vi "Process_single_meas.vi"(4 "Normalize?":bool, 6 "Calibration Constant (1/deg)":dbl, 7 "Magnet position":dbl, 8 "Magnetic Field (mT)":dbl, 9 "Actual Measurement":T2={"Elapsed Time (s)"=0.0, "Keithley"=0.0, "LockIn A"=[1.33515e-05, 1.14442e-05, 1.90736e-05, 41.634], "LockIn B"=[1.33515e-05, 1.14442e-05, 1.90736e-05, 41.634], "Dc intensity (V)"=0.0}) -> (3 "output cluster":T1)   [LabVIEW 2017]
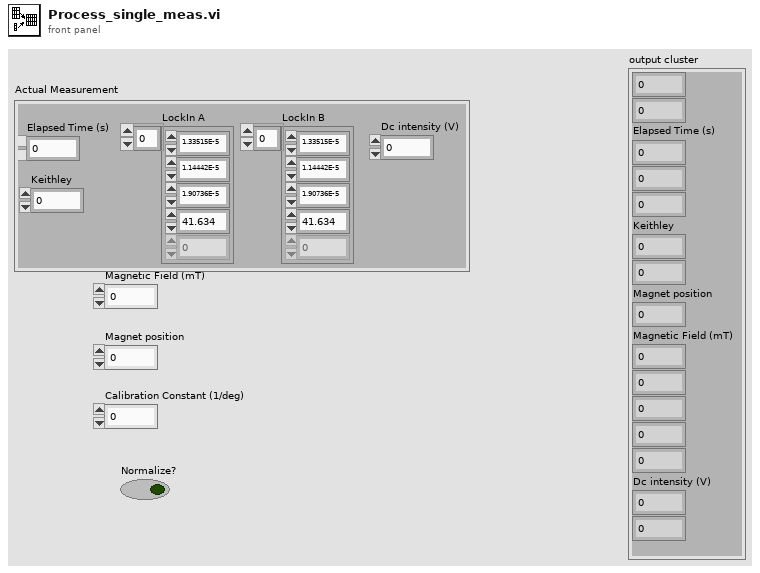
[diagram p1: front panel]
types:
  T1 = cluster{dbl, dbl, "Elapsed Time (s)":dbl, dbl, dbl, "Keithley":dbl, dbl, "Magnet position":dbl, "Magnetic Field (mT)":dbl, dbl, dbl, dbl, dbl, "Dc intensity (V)":dbl, dbl}
  T2 = cluster{"Elapsed Time (s)":dbl, "Keithley":dbl, "LockIn A":dbl[], "LockIn B":dbl[], "Dc intensity (V)":dbl}
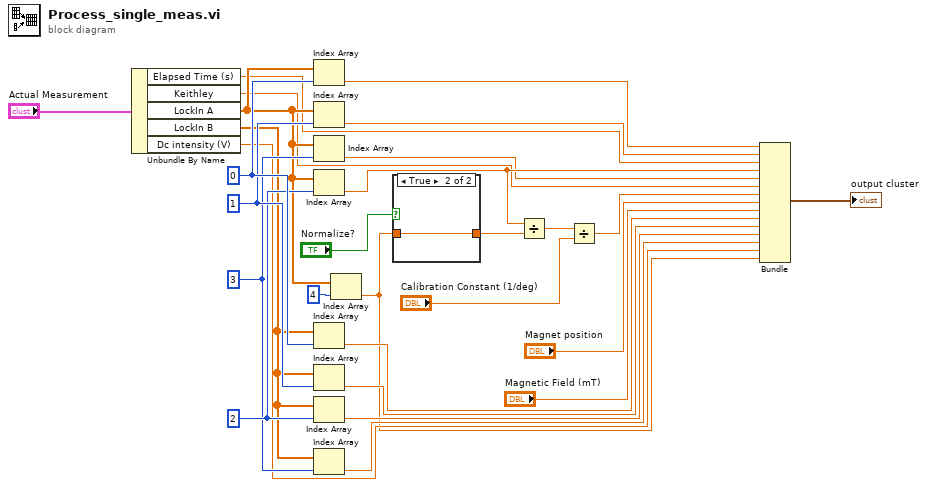
[diagram p0: block diagram]
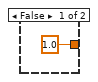
[diagram p2: hidden frame]
diagram:
  w23 = 3 ("index")
  w24 = 2 ("index")
  w25 = 1 ("index")
  w26 = 0 ("index")
  n1 = Unbundle By Name("Actual Measurement") -> ("Elapsed Time (s)"=w14:dbl, "Keithley"=w11:dbl, "LockIn A"=w19:dbl[], "LockIn B"=w22:dbl[], "Dc intensity (V)"=w3:dbl)
  n2 = Index Array(array=w19, index=w26) -> (element=w16:dbl)
  n3 = Index Array(array=w19, index=w25) -> (element=w15:dbl)
  n4 = Index Array(array=w19, index=w23) -> (element=w12:dbl)
  n5 = Index Array(array=w19, index=w24) -> (element=w13:dbl)
  n6 = Index Array(array=w22, index=w26) -> (element=w7:dbl)
  n7 = Index Array(array=w22, index=w25) -> (element=w6:dbl)
  n8 = Index Array(array=w22, index=w24) -> (element=w5:dbl)
  n9 = Index Array(array=w22, index=w23) -> (element=w4:dbl)
  n10 = Index Array(array=w19, index=4) -> (element=w2:dbl)
  n11 = case shown="True" "Normalize?" {
    tunnel: [1.0 ("Dc intensity (V)") w30] -> w21
    tunnel: w2 -> [_ w30]
    frame False {
    }
    frame True {
    }
  }
  n12 = Divide(x=w13, y=w21) -> (x/y=w27:dbl)
  n13 = Divide(x=w27, y="Calibration Constant (1/deg)") -> (x/y=w10:dbl)
  n14 = Bundle(w16, w15, "Elapsed Time (s)"=w14, w13, w12, "Keithley"=w11, w10, "Magnet position"="Magnet position", "Magnetic Field (mT)"="Magnetic Field (mT)", w7, w6, w5, w4, "Dc intensity (V)"=w3, w2) -> (→"output cluster":T1)  [unwired: 1 in]
